vi "FILE Read.vi"(0 "File Path (dialog if empty)":path, 1 "Pattern":string, 2 "Delimiter (Tab)":string="\t", 5 "File Type (text)":T1, 9 "Bytes to Read (-1: All)":i32=-1, 11 "Error In (no error)":errorcluster, 12 "Start Path":path) -> (4 "Spreadsheet Data (all)":string[][](array[string]), 6 "Spreadsheet Data (first col)":string[](array[string]), 8 "Spreadsheet Data (first row)":string[](array[string]), 10 "Output String":string, 13 "File Size (bytes)":i32, 14 "Opened File Path":path, 15 "Error Out":errorcluster)   [LabVIEW 2011]
doc: "This vi reads the file at the path specified, reads all the characters in the file, and then closes it. If spreadsheet file? is 'spreadsheet' then a spreadsheet convertion will be done and results output. Empty path causes a dialog to be opened for choosing the file to be read.\n\nnote: generally canceling out of all dialog boxes will not cause a file error to ocurr, only actual file errors will be flagged.\n\nThis vi was created by David Gianetto, contact me with any problems, questions, etc."
uses:
  Type Defs/FILE Type Enum.ctl
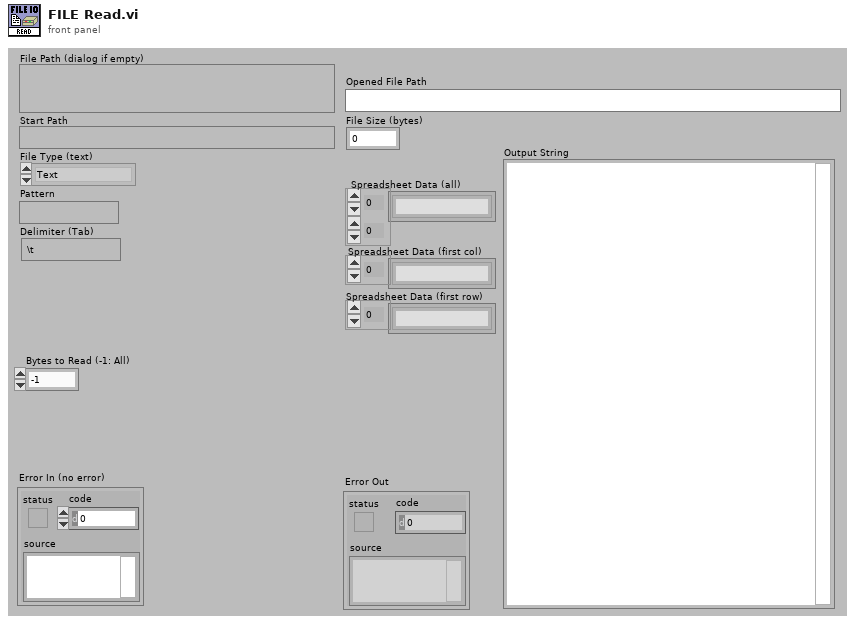
[diagram p1: front panel]
types:
  T1 = typedef "FILE Type Enum.ctl" = enum16{"Text", "Spreadsheet"}
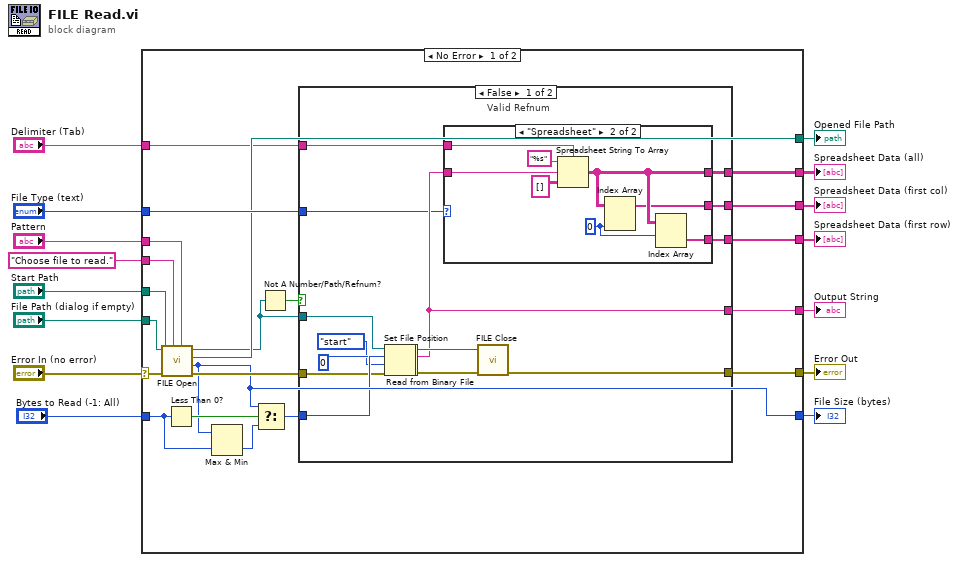
[diagram p0: block diagram]
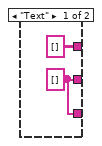
[diagram p2: hidden frame]
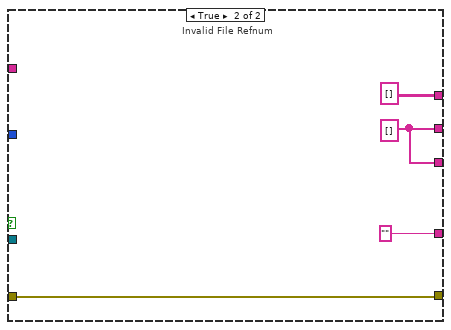
[diagram p3: hidden frame]
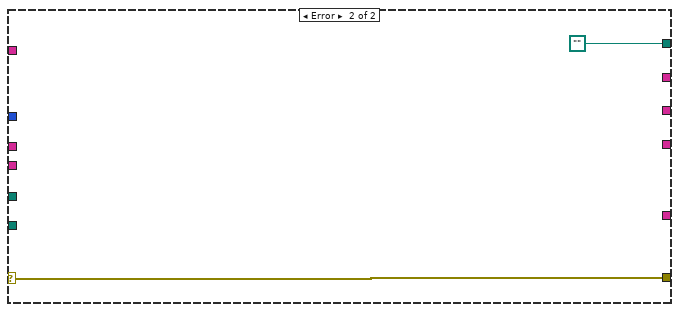
[diagram p4: hidden frame]
diagram:
  n1 = case shown="No Error" "Error In (no error)" {
    selector: "Error In (no error)" -> [w19 w67]
    tunnel: [w36 w67] -> w8
    tunnel: "File Type (text)" -> [w35 _]
    tunnel: [w34 _] -> w10
    tunnel: [w33 _] -> w11
    tunnel: [w32 _] -> w12
    tunnel: [w31 _] -> w13
    tunnel: "Choose file to read." ("prompt") -> [w29 _]
    tunnel: "File Path (dialog if empty)" -> [w28 _]
    tunnel: [w27 path ""] -> w7
    tunnel: "Start Path" -> [w26 _]
    tunnel: [w18 _] -> w5
    tunnel: "Pattern" -> [w25 _]
    tunnel: "Delimiter (Tab)" -> [w22 _]
    tunnel: "Bytes to Read (-1: All)" -> [w17 _]
    frame No Error {
      n2 = call "FILE Open.vi"("Pattern"=w25, "Dialog Prompt"=w29, "Error In (no error)"=w19, "Start path"=w26, "File Path (\" \")"=w28) -> ("Error Out"=w30:errorcluster, "Size (bytes)"=w18:i32, "Dup File Path"=w27:path, "Refnum"=w24:refnum<file>)  [unwired: 1 in, 2 out]
      n3 = Less Than 0?(x=w17) -> (x < 0?=w20:bool)
      n4 = Max & Min(x=w18, y=w17) -> (min(x,y)=w16:i32)  [unwired: 1 out]
      n5 = Select(t=w18, s=w20, f=w16) -> (s? t:f=w21:i32)
      n6 = Not A Number/Path/Refnum?(number/path/refnum=w24) -> (NaN/Path/Refnum?=w23:bool)
      n7 = case shown="False" w23 {
        tunnel: w21 -> [w52 _]
        tunnel: w24 -> [w49 _]
        tunnel: w30 -> [w48 w66]
        tunnel: [w45 ""] -> w31
        tunnel: [w44 w64] -> w32
        tunnel: [w43 string[][] [] ("array type (2D Dbl)")] -> w33
        tunnel: [w42 w64] -> w34
        tunnel: w35 -> [w41 _]
        tunnel: [w40 w66] -> w36
        tunnel: w22 -> [w39 _]
        frame False {
          # "Valid Refnum"
          n8 = Set File Position(offset (in bytes) (0)=0 ("pos offset (0)"), refnum=w49, from (0:start)=enum16{"start", "end", "current"}."start" ("pos mode (0:2)"), error in=w48) -> (refnum out=w38:refnum<file>, error out=w37:errorcluster)
          n9 = Read from Binary File(8:w37, 10:w52, 11:w38) -> (0:w47:errorcluster, 2:w45:string, 3:w46:refnum<file>)  [unwired: 4 out]
          n10 = case shown="\"Spreadsheet\"" w41 {
            tunnel: [w53 w62] -> w42
            tunnel: [string[][] [] ("array type (2D Dbl)") w60] -> w43
            tunnel: [w53 w59] -> w44
            tunnel: w45 -> [_ w57]
            tunnel: w39 -> [_ w55]
            frame "Text" {
              w53 = string[] [] ("array type (2D Dbl)")
            }
            frame "Spreadsheet" {
              w61 = 0
              n11 = Spreadsheet String To Array(delimiter (Tab)=w55, format string="%s", spreadsheet string=w57, array type (2D Dbl)=string[][] []) -> (array=w60:string[][])
              n12 = Index Array(array=w60, index (col)=w61) -> (element=w59:string[])  [unwired: 1 in]
              n13 = Index Array(array=w60, index (row)=w61) -> (element=w62:string[])  [unwired: 1 in]
            }
          }
          n14 = call "FILE Close.vi"("Error In (no error)"=w47, "Refnum"=w46) -> ("Error Out"=w40:errorcluster)  [unwired: 5 out]
        }
        frame True {
          w64 = string[] [] ("array type (2D Dbl)")
          # "Invalid File Refnum"
        }
      }
    }
    frame Error {
    }
  }
  "Output String" <- w13
  "Spreadsheet Data (all)" <- w11
  "Spreadsheet Data (first col)" <- w12
  "Spreadsheet Data (first row)" <- w10
  "Error Out" <- w8
  "Opened File Path" <- w7
  "File Size (bytes)" <- w5
